vi "Get Forces.vi"(10 "Device ID":i32, 11 "Force Table":dbl[][](array[numeric])) -> (2 "Dwell":dbl[](array[numeric]), 3 "Forces":dbl[](array[numeric]))   [LabVIEW 2015]
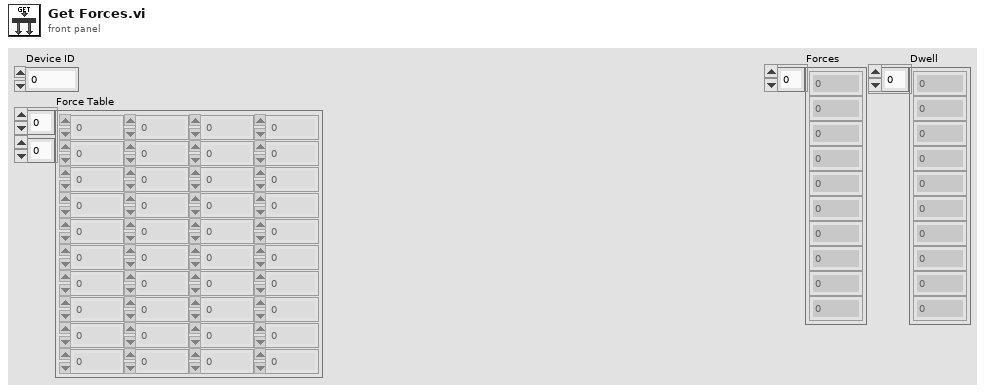
[diagram p1: front panel]
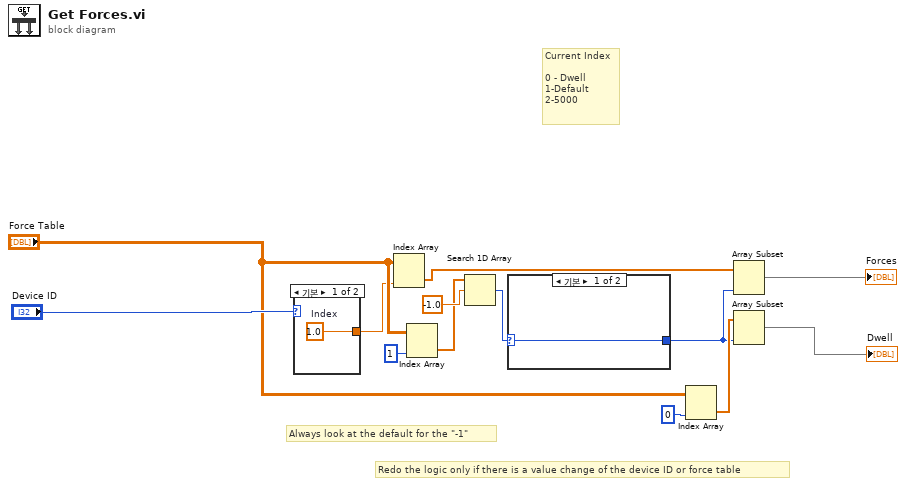
[diagram p0: block diagram]
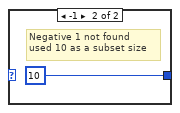
[diagram p2: hidden frame]
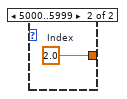
[diagram p3: hidden frame]
diagram:
  # "Always look at the default for the \"-1\""
  # "Redo the logic only if there is a value change of the device ID or force table"
  # "Current Index\n\n0 - Dwell\n1-Default\n2-5000"
  n1 = case shown="기본" "Device ID" {
    tunnel: [w14 w15] -> w10
    frame Default {
      w14 = 1.0  # Index
    }
    frame 5000..5999 {
      w15 = 2.0  # Index
    }
  }
  n2 = Index Array(array="Force Table", index (col)=w10) -> (element=w5:dbl[])  [unwired: 1 in]
  n3 = Index Array(array="Force Table", index (col)=1 ("disabled index (col)")) -> (element=w2:dbl[])  [unwired: 1 in]
  n4 = Search 1D Array(1D array=w2, element=-1.0) -> (index of element=w7:i32)  [unwired: 1 in]
  n5 = case shown="기본" w7 {
    selector: w7 -> [w16 _]
    tunnel: [w16 10 ("index of element")] -> w4
    frame Default {
    }
    frame -1 {
      # "Negative 1 not found\nused 10 as a subset size"
    }
  }
  n6 = Index Array(array="Force Table", index (col)=0 ("disabled index (col)")) -> (element=w6:dbl[])  [unwired: 1 in]
  n7 = Array Subset(array=w5, length=w4) -> (→"Forces":dbl[])  [unwired: 1 in]
  n8 = Array Subset(array=w6, length=w4) -> (→"Dwell":dbl[])  [unwired: 1 in]
